vi "Re_organise_RD_files.vi"() -> ()   [LabVIEW 2010]
uses:
  Controls/File_Selector_Type.ctl
  SW_Update_Tool/Sub_vis/Update_Global.vi
panel:
  out "Total Number":i32
  out "Current":i32
  out "Current":path
  out "No of unfound files":i32
  out "Array":string[](array[string])
  in  "File containing the raw data filenames":path
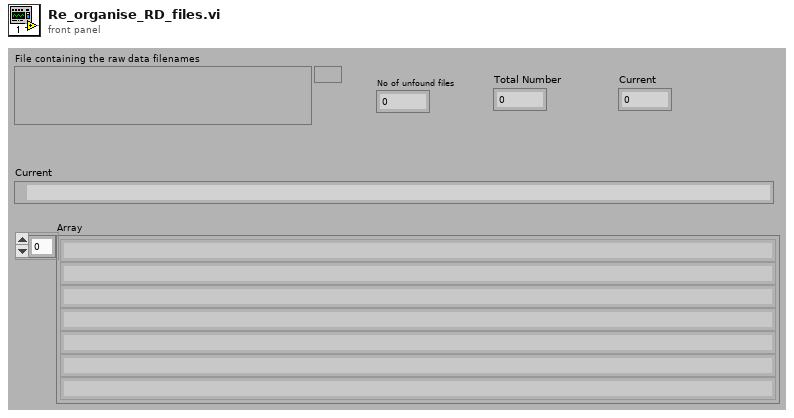
[diagram p1: front panel]
types:
  T1 = typedef "File_Selector_Type.ctl" = enum16{"The Selected File", "The Selected Folder", "Files containing the search string in the selected folder", "All files listed in selected file"}
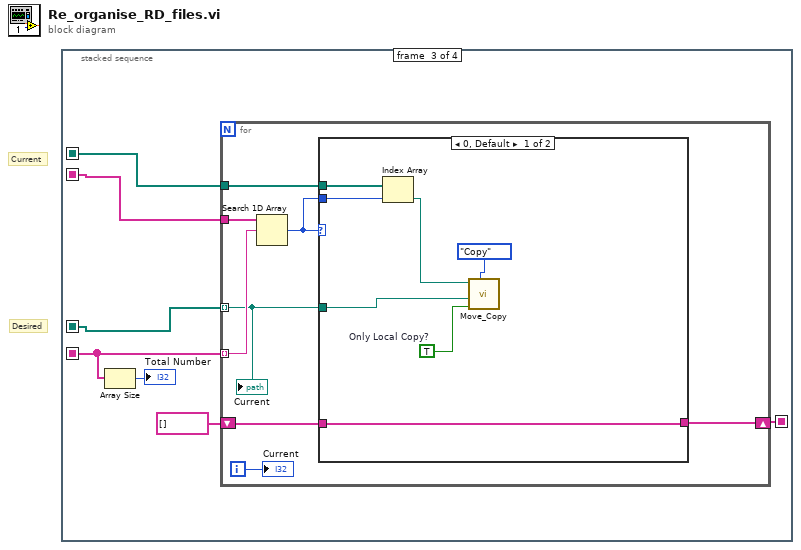
[diagram p0: block diagram]
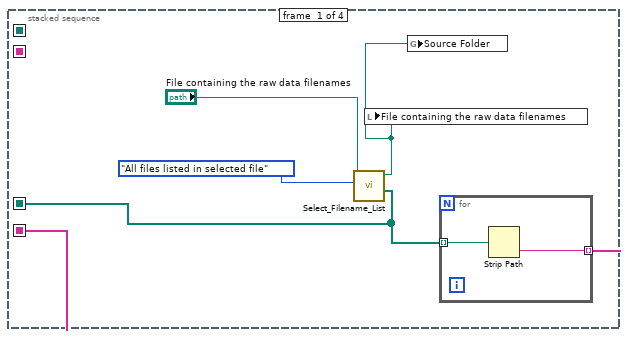
[diagram p2: hidden frame]
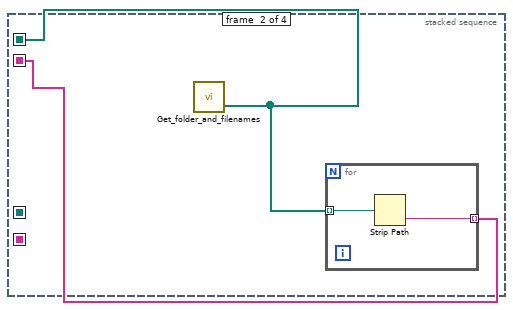
[diagram p3: hidden frame]
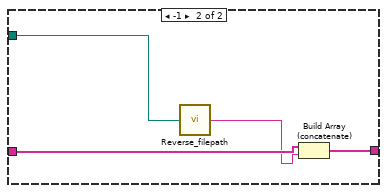
[diagram p4: hidden frame]
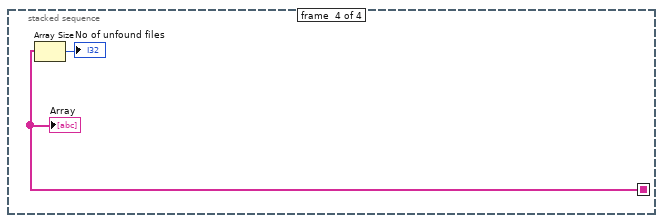
[diagram p5: hidden frame]
diagram:
  # "Current"
  # "Desired"
  n1 = stacked-sequence {
    seq-local: [_ w9 _ _] -> [_ _ w17 _]
    seq-local: [_ w8 _ _] -> [_ _ w18 _]
    seq-local: [w3 _ _ _] -> [_ _ w16 _]
    seq-local: [w2 _ _ _] -> [_ _ w13 _]
    seq-local: [_ _ w14 _] -> [_ _ _ w39]
    frame #0 {
      n2 = call "Select_Filename_List.vi"("At Dialog Prompt Post Process"=File_Selector_Type."All files listed in selected file", "Previous Choice"="File containing the raw data filenames") -> ("Selected files"=w3:path[], "Choosen path"=w1:path)  [unwired: 4 in, 1 out]
      n3 = local write "File containing the raw data filenames"(w1) -> ()
      n4 = global write "Update_Global.vi" "Source Folder"(w1) -> ()
      n5 = for {
        tunnel: w3 -> [w7] mode=indexing
        tunnel: [w6] -> w2 mode=indexing
        n6 = Strip Path(path=w7) -> (name=w6:string)  [unwired: 1 out]
      }
    }
    frame #1 {
      n7 = call "Get_folder_and_filenames.vi"() -> ("Files"=w9:path[])  [unwired: 1 in, 1 out]
      n8 = for {
        tunnel: w9 -> [w11] mode=indexing
        tunnel: [w10] -> w8 mode=indexing
        n9 = Strip Path(path=w11) -> (name=w10:string)  [unwired: 1 out]
      }
    }
    frame #2 {
      n10 = Array Size(array=w13) -> (size(s)=→"Total Number":i32)
      n11 = for {
        tunnel: w18 -> [w26]
        tunnel: w13 -> [w25] mode=indexing
        tunnel: w17 -> [w23]
        tunnel: w16 -> [w22] mode=indexing
        shift-right: [w20] -> w14
        shift-left: string[] [] -> [w21]
        i -> [w19]
        n12 = Search 1D Array(1D array=w26, element=w25) -> (index of element=w24:i32)  [unwired: 1 in]
        n13 = case shown="0, Default" w24 {
          tunnel: w24 -> [w33 _]
          tunnel: w23 -> [w32 _]
          tunnel: w22 -> [w29 w35]
          tunnel: w21 -> [w28 w37]
          tunnel: [w28 w36] -> w20
          frame 0, Default {
            w27 = TRUE  # Only Local Copy?
            n14 = Index Array(array=w32, index=w33) -> (element=w30:path)
            n15 = call "Move_Copy.vi"("Mode"=enum16{"Move", "Copy"}."Copy", "Only Local Copy?"=w27, "target path"=w29, "source path"=w30) -> ()  [unwired: 3 in]
          }
          frame -1 {
            n16 = call "Reverse_filepath.vi"("Filename"=w35) -> ("Reversed Filepath"=w34:string)
            n17 = Build Array (concatenate)(w37, w34) -> (w36:string[])
          }
        }
        "Current" <- w22
        "Current" <- w19
      }
    }
    frame #3 {
      n18 = Array Size(array=w39) -> (size(s)=→"No of unfound files":i32)
      "Array" <- w39
    }
  }
